vi "Elevator Logic Test.vi"() -> ()   [LabVIEW 2014]
uses:
  <vilib>/addons/control/pid/NI_PID_pid.lvlib
  <vilib>/addons/control/pid/pid.llb/PID Output Rate Limiter (DBL).vi
  Robot Code/Elevator/Elevator Presets.ctl
panel:
  in  "Presets":T1
  in  "Sim speed":dbl=1.0 format="%.2f"
  in  "Command":T2(ring)
  in  "High IR":bool
  in  "Low IR":bool
  out "Ejector Piston":bool
  out "Lift Plates":bool
  out "Level":dbl(slide) scale=0.0..10.0
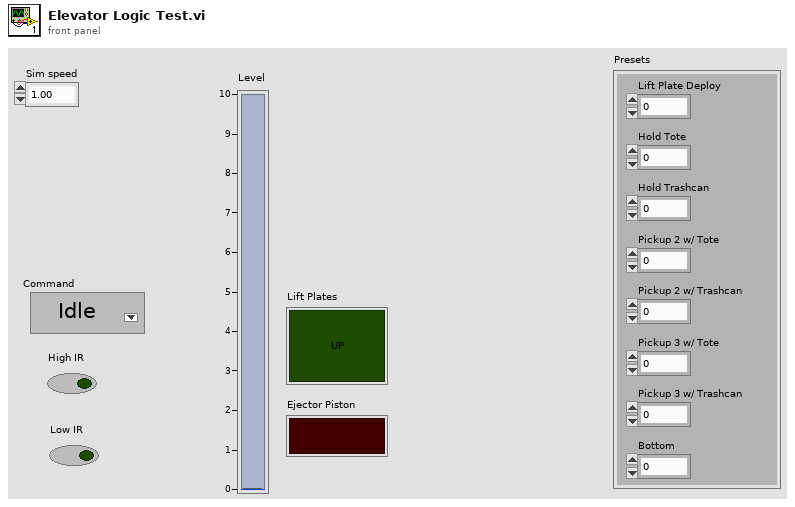
[diagram p1: front panel]
types:
  T1 = typedef "Elevator Presets.ctl" = cluster{"Hold Tote":dbl, "Hold Trashcan":dbl, "Pickup 2 w/ Tote":dbl, "Pickup 2 w/ Trashcan":dbl, "Pickup 3 w/ Tote":dbl, "Pickup 3 w/ Trashcan":dbl, "Lift Plate Deploy":dbl, "Bottom":dbl}
  T2 = enum16{"Idle", "Load 1", "Load 2", "Load 3", "Drop Stack", "Eject Stack"}
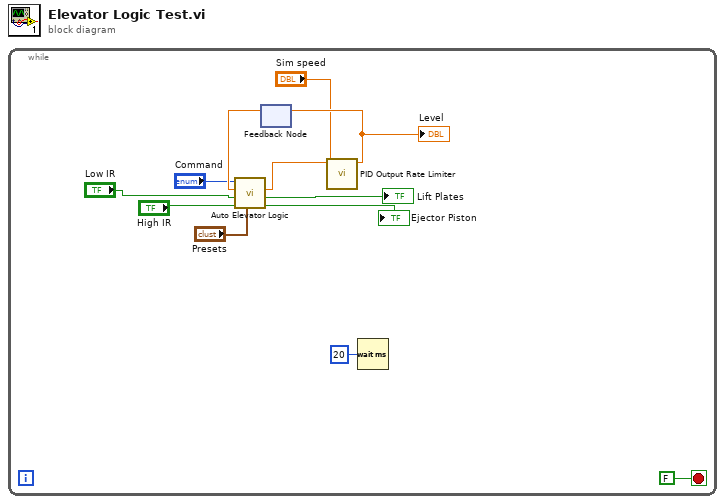
[diagram p0: block diagram]
diagram:
  n1 = while {
    stop <- FALSE stop-if-true
    n2 = feedback #1() -> (w9:dbl)  [unwired: 1 in]
    n3 = call "Auto Elevator Logic.vi"("Presets"="Presets", "High IR"="High IR", "Low IR"="Low IR", "Current Position"=w9, "Command"="Command") -> ("Ejector Piston"=→"Ejector Piston":bool, "Lift Plates Deploy"=→"Lift Plates":bool, "Position Out"=w10:dbl)  [unwired: 4 in]
    n4 = call-poly <vilib>:"PID Output Rate Limiter.vi"("output rate (EGU/min)"="Sim speed", "input (controller output)"=w10) -> ("output"=w4:dbl)  [unwired: 6 in, 1 out]
    "Level" <- w4
    n5 = feedback-in #1(w4) -> ()
    n6 = Wait (ms)(milliseconds to wait=u32 20) -> ()  [unwired: 1 out]
  }
